vi "Scaffold Saveas.vi"(11 "Item Ref":T1) -> ()   [LabVIEW 2020, in "Negentropic IDE.lvlib"]
uses:
  Negentropic IDE.lvlib
  <resource>/Framework/Providers/API/ItemRef.ctl
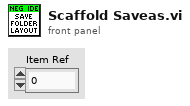
[diagram p1: front panel]
types:
  T1 = typedef "ItemRef.ctl" = u64
  T2 = typedef "Negentropic IDE.lvlib/Folder Config.ctl" = cluster{"Path":string, "Scope":T3}
  T3 = typedef "Negentropic IDE.lvlib/Scope.ctl" = enum32{"invalid scope", "public", "private", "protected", "community"}
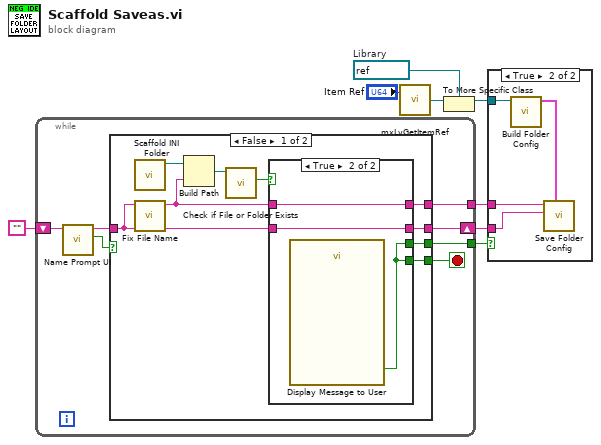
[diagram p0: block diagram]
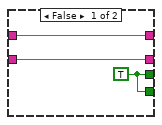
[diagram p2: hidden frame]
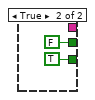
[diagram p3: hidden frame]
diagram:
  w6 = refnum<vi> refnum  # Library
  n1 = while {
    tunnel: [w13] -> w4
    tunnel: [w10] -> w2
    shift-right: [w11] -> w3
    shift-left: "" -> [w9]
    stop <- w12 stop-if-true
    n2 = call "Name Prompt UI.vi"("Initial Name (Empty)"=w9) -> ("Cancelled"=w15:bool, "Name"=w14:string)  [unwired: 9 in]
    n3 = case shown="False" w15 {
      tunnel: w14 -> [w19 _]
      tunnel: [w20 FALSE ("Yes")] -> w13
      tunnel: [w21 TRUE ("Yes")] -> w12
      tunnel: [w17 _] -> w11
      tunnel: [w16 _] -> w10
      frame False {
        n4 = call "Scaffold INI Folder.vi"() -> ("Scaffold INI Folder"=w24:path)  [unwired: 10 in, 1 out]
        n5 = call "Fix File Name.vi"("Config Name"=w19) -> ("File Name"=w18:string)  [unwired: 10 in]
        n6 = Build Path(base path=w24, name or relative path=w18) -> (appended path=w23:path)
        n7 = call <vilib>:"Check if File or Folder Exists.vi"("path"=w23) -> ("file or folder exists?"=w22:bool)  [unwired: 8 in, 2 out]
        n8 = case shown="True" w22 {
          tunnel: [w25 w30] -> w21
          tunnel: [w25 w30] -> w20
          tunnel: w19 -> [w27 w29]
          tunnel: w18 -> [w26 w28]
          tunnel: [w27 w29] -> w17
          tunnel: [w26 w28] -> w16
          frame False {
            w25 = TRUE ("Yes")
          }
          frame True {
            n9 = call "Display Message to User"() -> ("Yes"=w30:bool)  [unwired: 10 in, 1 out]
          }
        }
      }
      frame True {
      }
    }
  }
  n10 = call <resource>:"mxLvGetItemRef.vi"("Item"="Item Ref") -> ("Item Refnum"=w7:refnum<vi>)  [unwired: 1 in, 2 out]
  n11 = To More Specific Class(target class=w6, reference=w7) -> (specific class reference=w5:refnum<vi>)  [unwired: 1 in, 1 out]
  n12 = case shown="True" w4 {
    tunnel: w5 -> [_ w36]
    tunnel: w3 -> [_ w33]
    tunnel: w2 -> [_ w34]
    frame False {
    }
    frame True {
      n13 = call "Build Folder Config.vi"("Library"=w36) -> ("Folders"=w35:T2[])  [unwired: 10 in]
      n14 = call "Save Folder Config.vi"("Folder Config"=w35, "Name"=w33, "INI Filename"=w34) -> ()  [unwired: 8 in, 1 out]
    }
  }
